vi "commandClusterRebuilder.vi"() -> ()   [LabVIEW 2018]
uses:
  PololuCommandDescriptor.ctl
  TicCommandType.ctl
panel:
  out "CommandDescriptorArray 2":T1[](array[typedef])
  in  "CommandDescriptorArray":T3(array[cluster])=[{"PololuCommand"="SetTargetPosition", "Mnemonic"="à", "CommandType"=enum."32-bitWrite", "Min"=-2147483648, "Max"=2147483647}, {"PololuCommand"="SetTargetVelocity", "Mnemonic"="ã", "CommandType"=enum."32-bitWrite", "Min"=-500000000, "Max"=500000000}, {"PololuCommand"="HaltSetPosition", "Mnemonic"="ì", "CommandType"=enum."32-bitWrite", "Min"=-2147483648, "Max"=2147483647}, {"PololuCommand"="HaltHold", "Mnemonic"="‰", "CommandType"=enum."Quick", "Min"=0, "Max"=0}, {"PololuCommand"="ResetTimeout", "Mnemonic"="Œ", "CommandType"=enum."Quick", "Min"=0, "Max"=0}, {"PololuCommand"="De-energize", "Mnemonic"="†", "CommandType"=enum."Quick", "Min"=0, "Max"=0}, {"PololuCommand"="Energize", "Mnemonic"="…", "CommandType"=enum."Quick", "Min"=0, "Max"=0}, {"PololuCommand"="ExitSafeStart", "Mnemonic"="ƒ", "CommandType"=enum."Quick", "Min"=0, "Max"=0}, {"PololuCommand"="EnterSafeStart", "Mnemonic"="", "CommandType"=enum."Quick", "Min"=0, "Max"=0}, {"PololuCommand"="Reset", "Mnemonic"="°", "CommandType"=enum."Quick", "Min"=0, "Max"=0}, {"PololuCommand"="ClearDriverError", "Mnemonic"="Š", "CommandType"=enum."Quick", "Min"=0, "Max"=0}, {"PololuCommand"="SetMaxSpeed", "Mnemonic"="æ", "CommandType"=enum."32-bitWrite", "Min"=0, "Max"=500000000}, {"PololuCommand"="SetStartSpeed", "Mnemonic"="å", "CommandType"=enum."32-bitWrite", "Min"=0, "Max"=500000000}, {"PololuCommand"="SetMaxAcc", "Mnemonic"="ê", "CommandType"=enum."32-bitWrite", "Min"=100, "Max"=2147483647}, {"PololuCommand"="SetMaxDec", "Mnemonic"="é", "CommandType"=enum."32-bitWrite", "Min"=0, "Max"=2147483647}, {"PololuCommand"="SetStepMode", "Mnemonic"="”", "CommandType"=enum."7-bitWrite", "Min"=0, "Max"=5}, {"PololuCommand"="SetCurrLim", "Mnemonic"="‘", "CommandType"=enum."7-bitWrite", "Min"=0, "Max"=124}, {"PololuCommand"="SetDecayMode", "Mnemonic"="’", "CommandType"=enum."7-bitWrite", "Min"=0, "Max"=4}, {"PololuCommand"="GetVar", "Mnemonic"="¡", "CommandType"=enum."BlockRead", "Min"=0, "Max"=81}, {"PololuCommand"="GetVarClrErr", "Mnemonic"="¢", "CommandType"=enum."BlockRead", "Min"=0, "Max"=81}, {"PololuCommand"="GetSetting", "Mnemonic"="¨", "CommandType"=enum."BlockRead", "Min"=0, "Max"=94}]
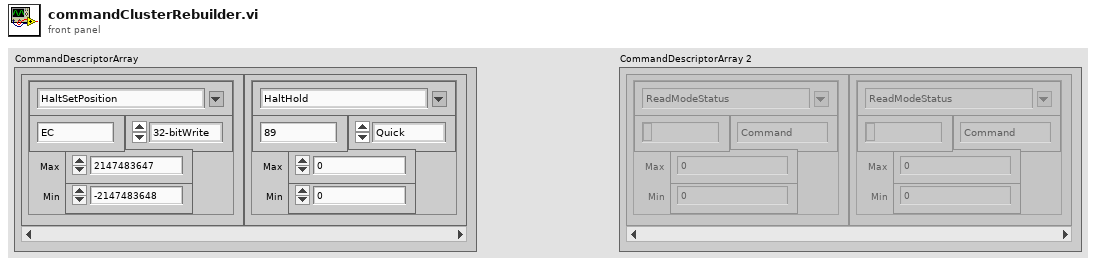
[diagram p1: front panel]
types:
  T1 = typedef "PololuCommandDescriptor.ctl" = cluster{"PololuCommand":string, "Mnemonic":string, "CommandType":T2, "Min":i32, "Max":i32}
  T2 = typedef "TicCommandType.ctl" = enum16{"Command", "7-bitWrite", "32-bitWrite", "BlockRead"}
  T3 = cluster{"PololuCommand":string, "Mnemonic":string, "CommandType":enum16{"Quick", "7-bitWrite", "32-bitWrite", "BlockRead"}, "Min":i32, "Max":i32}[]
  T4 = enum16{"Quick", "7-bitWrite", "32-bitWrite", "BlockRead"}
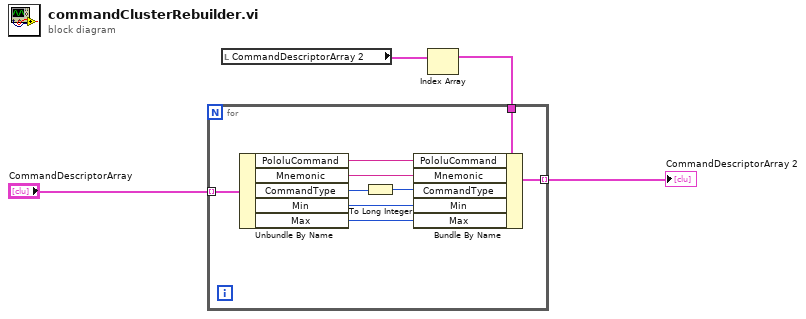
[diagram p0: block diagram]
diagram:
  n1 = local read "CommandDescriptorArray 2"() -> (w2:T1[])
  n2 = Index Array(array=w2) -> (element=w1:T1)  [unwired: 1 in]
  n3 = for {
    tunnel: [w13] -> w4 mode=indexing
    tunnel: "CommandDescriptorArray" -> [w11] mode=indexing
    tunnel: w1 -> [w12]
    n4 = Unbundle By Name(w11) -> ("PololuCommand"=w10:string, "Mnemonic"=w9:string, "CommandType"=w6:T4, "Min"=w8:i32, "Max"=w7:i32)
    n5 = To Long Integer(number=w6) -> (32bit integer=w5:i32)
    n6 = Bundle By Name(cluster=w12, "PololuCommand"=w10, "Mnemonic"=w9, "CommandType"=w5, "Min"=w8, "Max"=w7) -> (w13:T1)
  }
  "CommandDescriptorArray 2" <- w4
